vi "GetSetWindowPosition.vi"(8 "error in":errorcluster, 10 "Read":bool, 11 "ViRef":refnum<vi>) -> (0 "error out":errorcluster)   [LabVIEW 2018, in "GUI.lvclass"]
uses:
  GUI.lvclass
  <vilib>/Utility/miscctls.llb/LVRectTypeDef.ctl
  1e420645-825f-4e80-8f0e-5784f8e70d06.vi
  5344164c-4383-4e6f-abf5-59efef7f4b2c.vi
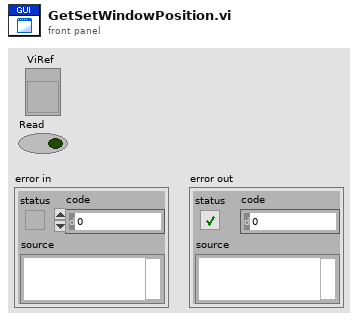
[diagram p1: front panel]
types:
  T1 = enum16{"open", "replace", "create", "open or create", "replace or create", "replace or create with confirmation"}
  T2 = typedef "LVRectTypeDef.ctl" = cluster{"Left":i16, "Top":i16, "Right":i16, "Bottom":i16}
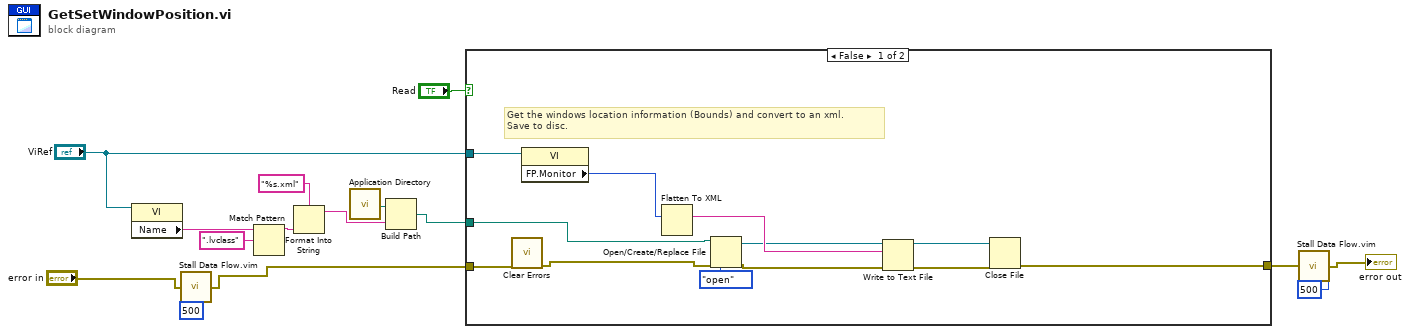
[diagram p0: block diagram]
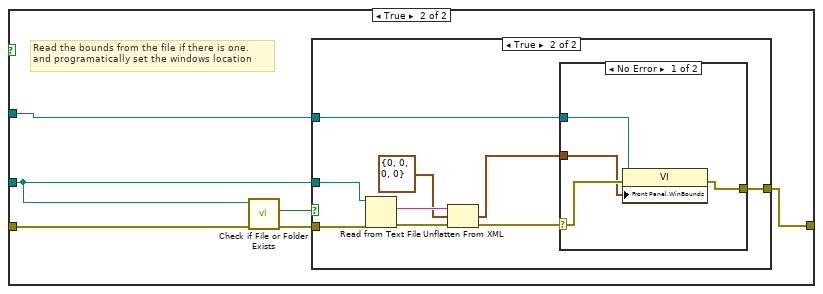
[diagram p2: hidden frame]
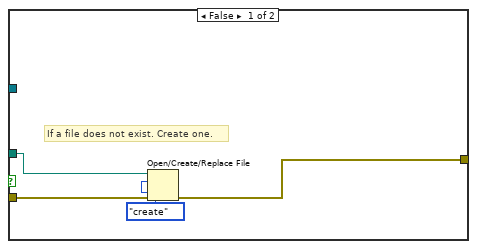
[diagram p3: hidden frame]
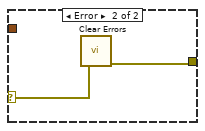
[diagram p4: hidden frame]
diagram:
  n1 = property class="VI"(reference="ViRef") -> ("Name"=w9:string)  [unwired: 1 in, 2 out]
  n2 = call "Stall Data Flow.vim"("value in"="error in", "milliseconds to wait"=u32 500) -> ("value out"=w4:errorcluster)  [unwired: 1 out]
  n3 = Match Pattern(string=w9, regular expression=".lvclass") -> (before substring=w7:string)  [unwired: 1 in, 3 out]
  n4 = Format Into String(format string="%s.xml", w7) -> (resulting string=w13:string)  [unwired: 2 in, 1 out]
  n5 = call <vilib>:"Application Directory.vi"() -> ("Application Directory"=w12:path)
  n6 = Build Path(base path=w12, name or relative path=w13) -> (appended path=w10:path)
  n7 = case shown="False" "Read" {
    tunnel: [w19 w30] -> w3
    tunnel: w4 -> [w18 w32]
    tunnel: "ViRef" -> [w27 w29]
    tunnel: w10 -> [w24 w28]
    frame False {
      # "Get the windows location information (Bounds) and convert to an xml. \nSave to disc."
      n8 = call <vilib>:"Clear Errors.vi"("error in (no error)"=w18) -> ("error out"=w17:errorcluster)  [unwired: 5 in, 1 out]
      n9 = property class="VI"(reference=w27) -> ("FP.Monitor"=w26:u16)  [unwired: 1 in, 2 out]
      n10 = Flatten To XML(anything=w26) -> (xml string=w25:string)
      n11 = Open/Create/Replace File(file path (use dialog)=w24, error in=w17, operation (0:open)=T1."open") -> (refnum out=w22:refnum<file>, error out=w16:errorcluster)  [unwired: 3 in, 1 out]
      n12 = Write to Text File(file (use dialog)=w22, text=w25, error in=w16) -> (refnum out=w21:refnum<file>, error out=w20:errorcluster)  [unwired: 1 in, 1 out]
      n13 = Close File(refnum=w21, error in=w20) -> (error out=w19:errorcluster)  [unwired: 1 out]
    }
    frame True {
      # "Read the bounds from the file if there is one. \nand programatically set the windows location"
      n14 = call <vilib>:"Check if File or Folder Exists.vi"("error in (no error)"=w32, "path"=w28) -> ("error out"=w31:errorcluster, "file or folder exists?"=w33:bool)  [unwired: 7 in, 1 out]
      n15 = case shown="True" w33 {
        tunnel: w28 -> [w37 w46]
        tunnel: [w35 w38] -> w30
        tunnel: w31 -> [w34 w45]
        tunnel: w29 -> [_ w41]
        frame False {
          # "If a file does not exist. Create one."
          n16 = Open/Create/Replace File(file path (use dialog)=w37, error in=w34, operation (0:open)=T1."create") -> (error out=w35:errorcluster)  [unwired: 3 in, 2 out]
        }
        frame True {
          n17 = Read from Text File(file (use dialog)=w46, error in=w45) -> (text=w44:string, error out=w42:errorcluster)  [unwired: 2 in, 2 out]
          n18 = Unflatten From XML(xml string=w44, type=T2 {"Left"=0, "Top"=0, "Right"=0, "Bottom"=0} ("Front Panel Window:Window Bounds"), error in (no error)=w42) -> (value=w39:T2, error out=w40:errorcluster)
          n19 = case shown="No Error" w40 {
            selector: w40 -> [w50 w52]
            tunnel: w39 -> [w48 _]
            tunnel: [w49 w51] -> w38
            tunnel: w41 -> [w47 _]
            frame No Error {
              n20 = property class="VI"(reference=w47, error in=w50, "Front Panel.WinBounds"=w48) -> (error out=w49:errorcluster)  [unwired: 1 out]
            }
            frame Error {
              n21 = call <vilib>:"Clear Errors.vi"("error in (no error)"=w52) -> ("error out"=w51:errorcluster)  [unwired: 5 in, 1 out]
            }
          }
        }
      }
    }
  }
  n22 = call "Stall Data Flow.vim"("value in"=w3, "milliseconds to wait"=u32 500) -> ("value out"=→"error out":errorcluster)  [unwired: 1 out]
